vi "Shutdown.vi"(8 "error in (no error)":errorcluster, 11 "DAQ":refnum<class "DAQ.lvclass">) -> (0 "error out":errorcluster, 3 "DAQ":refnum<class "DAQ.lvclass">)   [LabVIEW 2017, in "DAQ.lvclass"]
doc: "Developed by Kevin Thompson\nkevin@thompsonengineering.net\n\nCopyright 2018-2020\nThompson Engineering, LLC"
uses:
  DAQ.lvclass
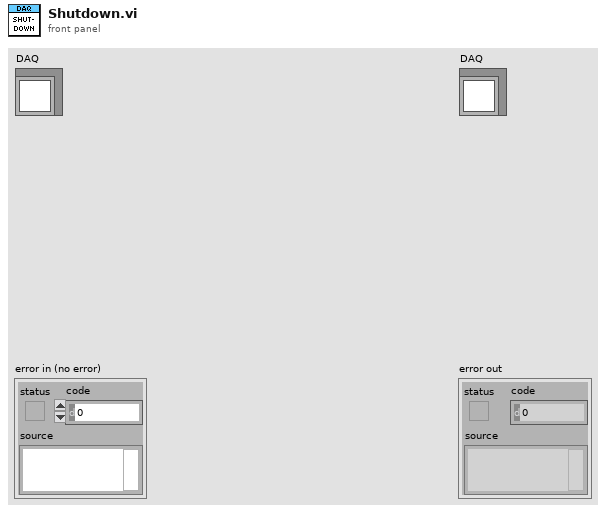
[diagram p1: front panel]
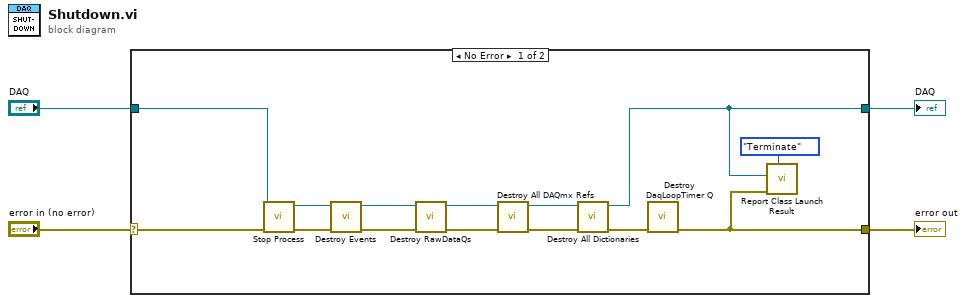
[diagram p0: block diagram]
diagram:
  n1 = case shown="No Error" "error in (no error)" {
    selector: "error in (no error)" -> [w15 w20]
    tunnel: [w6 w20] -> w3
    tunnel: [w5 w19] -> w1
    tunnel: "DAQ" -> [w13 w19]
    frame No Error {
      n2 = call "Stop Process.vi"("error in (no error)"=w15, "DAQ"=w13) -> ("error out"=w14:errorcluster, "DAQ"=w12:refnum<class "DAQ.lvclass">)  [unwired: 8 in]
      n3 = call "Destroy Events.vi"("error in (no error)"=w14, "DAQ"=w12) -> ("error out"=w11:errorcluster, "DAQ"=w10:refnum<class "DAQ.lvclass">)  [unwired: 8 in]
      n4 = call "Destroy RawDataQs.vi"("error in (no error)"=w11, "DAQ"=w10) -> ("error out"=w8:errorcluster, "DAQ"=w9:refnum<class "DAQ.lvclass">)  [unwired: 8 in]
      n5 = call "Destroy All DAQmx Refs.vi"("error in (no error)"=w8, "DAQ"=w9) -> ("error out"=w17:errorcluster, "DAQ"=w18:refnum<class "DAQ.lvclass">)  [unwired: 8 in]
      n6 = call "Destroy All Dictionaries.vi"("error in (no error)"=w17, "DAQ"=w18) -> ("error out"=w16:errorcluster, "DAQ"=w5:refnum<class "DAQ.lvclass">)  [unwired: 8 in]
      n7 = call "Destroy DaqLoopTimer Q.vi"("error in (no error)"=w16) -> ("error out"=w6:errorcluster)  [unwired: 9 in, 1 out]
      n8 = call "Report Class Launch Result.vi"("Object"=w5, "error in (no error)"=w6, "Mode (Launch)"=enum16{"Launch", "Terminate"}."Terminate") -> ()  [unwired: 7 in, 1 out]
    }
    frame Error {
    }
  }
  "error out" <- w3
  "DAQ" <- w1
